vi "Axis Property to Cluster.vi"(11 "Axis Property Array In":T1[](array[typedef])) -> (3 "Axis Property Out":T2)   [LabVIEW 2020, in "3D Plot.lvclass"]
uses:
  <vilib>/Math Plots/3D Math Plots/3D Plot/3D Plot/3D Plot.lvclass
  <vilib>/Math Plots/3D Math Plots/3D Plot/3D Plot/Typedef/Axis Property.ctl
  <vilib>/Math Plots/3D Math Plots/3D Plot/3D Plot/Typedef/Caption Property.ctl
  <vilib>/Math Plots/3D Math Plots/3D Plot/3D Plot/Typedef/Label Property.ctl
  <vilib>/Math Plots/3D Math Plots/3D Plot/3D Plot/Typedef/Range Property.ctl
  <vilib>/Math Plots/3D Math Plots/3D Plot/3D Plot/Typedef/Range Clusters.ctl
  <vilib>/Math Plots/3D Math Plots/3D Plot/3D Plot/Typedef/Grid Property.ctl
  <vilib>/Math Plots/3D Math Plots/3D Plot/3D Plot/Typedef/Tick Property.ctl
  <vilib>/Math Plots/3D Math Plots/3D Plot/3D Plot/Typedef/Axis Property Array Element.ctl
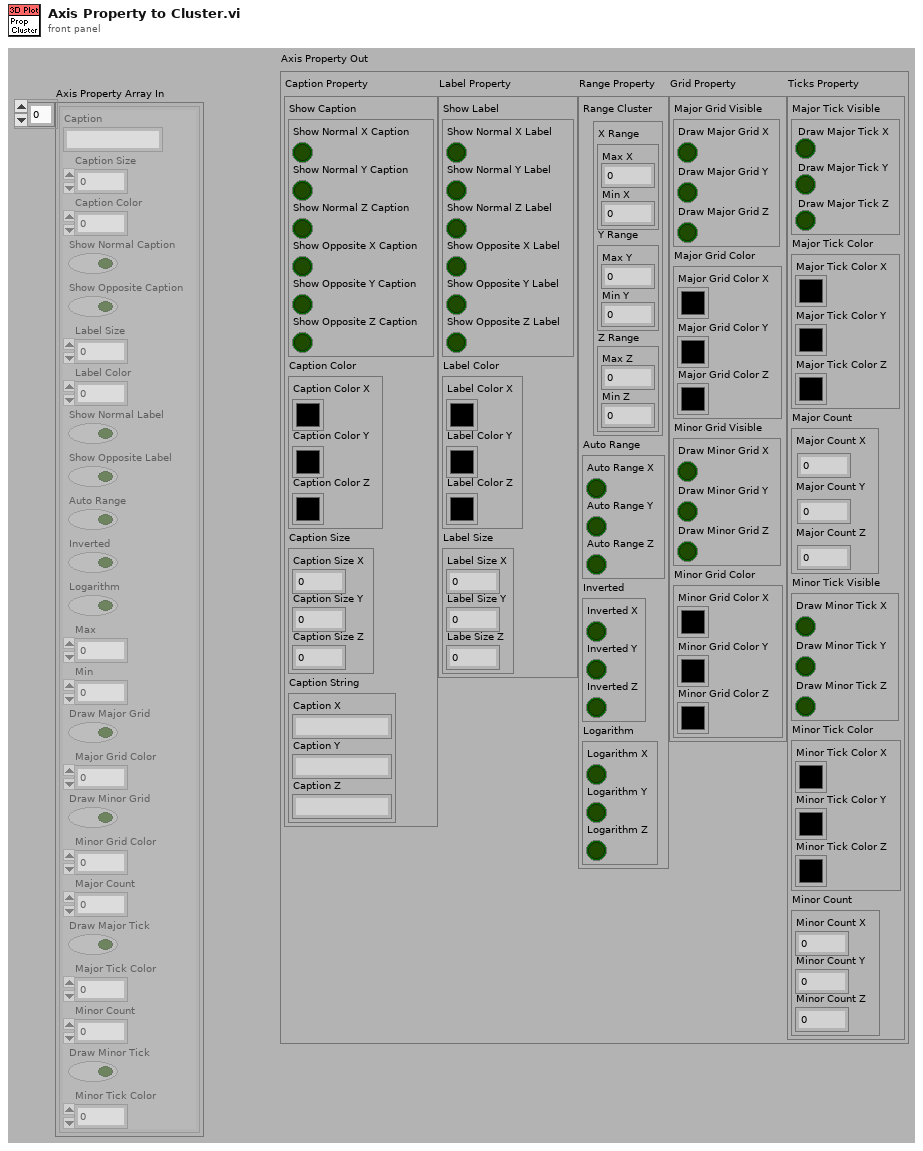
[diagram p1: front panel]
types:
  T1 = typedef "3D Plot.lvclass/Axis Property Array Element.ctl" = cluster{"Caption":string, "Caption Size":u16, "Caption Color":u32, "Show Normal Caption":bool, "Show Opposite Caption":bool, "Label Size":u16, "Label Color":u32, "Show Normal Label":bool, "Show Opposite Label":bool, "Auto Range":bool, "Inverted":bool, "Logarithm":bool, "Max":sgl, "Min":sgl, "Draw Major Grid":bool, "Major Grid Color":u32, "Draw Minor Grid":bool, "Minor Grid Color":u32, "Major Count":u16, "Draw Major Tick":bool, "Major Tick Color":u32, "Minor Count":u16, "Draw Minor Tick":bool, "Minor Tick Color":u32}
  T2 = typedef "3D Plot.lvclass/Axis Property.ctl" = cluster{"Caption Property":T3, "Label Property":T4, "Range Property":T5, "Grid Property":T7, "Ticks Property":T8}
  T3 = typedef "3D Plot.lvclass/Caption Property.ctl" = cluster{"Show Caption":cluster{"Show Normal X Caption":bool, "Show Normal Y Caption":bool, "Show Normal Z Caption":bool, "Show Opposite X Caption":bool, "Show Opposite Y Caption":bool, "Show Opposite Z Caption":bool}, "Caption Color":cluster{"Caption Color X":u32, "Caption Color Y":u32, "Caption Color Z":u32}, "Caption Size":cluster{"Caption Size X":u16, "Caption Size Y":u16, "Caption Size Z":u16}, "Caption String":cluster{"Caption X":string, "Caption Y":string, "Caption Z ":string}}
  T4 = typedef "3D Plot.lvclass/Label Property.ctl" = cluster{"Show Label":cluster{"Show Normal X Label":bool, "Show Normal Y Label":bool, "Show Normal Z Label":bool, "Show Opposite X Label":bool, "Show Opposite Y Label":bool, "Show Opposite Z Label":bool}, "Label Color":cluster{"Label Color X":u32, "Label Color Y":u32, "Label Color Z":u32}, "Label Size":cluster{"Label Size X":u16, "Label Size Y":u16, "Labe Size Z":u16}}
  T5 = typedef "3D Plot.lvclass/Range Property.ctl" = cluster{"Range Cluster":T6, "Auto Range":cluster{"Auto Range X":bool, "Auto Range Y":bool, "Auto Range Z":bool}, "Inverted":cluster{"Inverted X":bool, "Inverted Y":bool, "Inverted Z":bool}, "Logarithm":cluster{"Logarithm X":bool, "Logarithm Y":bool, "Logarithm Z":bool}}
  T6 = typedef "3D Plot.lvclass/Range Clusters.ctl" = cluster{"X Range":cluster{"Max X":sgl, "Min X":sgl}, "Y Range":cluster{"Max Y":sgl, "Min Y":sgl}, "Z Range":cluster{"Max Z":sgl, "Min Z":sgl}}
  T7 = typedef "3D Plot.lvclass/Grid Property.ctl" = cluster{"Major Grid Visible":cluster{"Draw Major Grid X":bool, "Draw Major Grid Y":bool, "Draw Major Grid Z":bool}, "Major Grid Color":cluster{"Major Grid Color X":u32, "Major Grid Color Y":u32, "Major Grid Color Z":u32}, "Minor Grid Visible":cluster{"Draw Minor Grid X":bool, "Draw Minor Grid Y":bool, "Draw Minor Grid Z":bool}, "Minor Grid Color":cluster{"Minor Grid Color X":u32, "Minor Grid Color Y":u32, "Minor Grid Color Z":u32}}
  T8 = typedef "3D Plot.lvclass/Tick Property.ctl" = cluster{"Major Tick Visible":cluster{"Draw Major Tick X":bool, "Draw Major Tick Y":bool, "Draw Major Tick Z":bool}, "Major Tick Color":cluster{"Major Tick Color X":u32, "Major Tick Color Y":u32, "Major Tick Color Z":u32}, "Major Count":cluster{"Major Count X":u16, "Major Count Y":u16, "Major Count Z":u16}, "Minor Tick Visible":cluster{"Draw Minor Tick X":bool, "Draw Minor Tick Y":bool, "Draw Minor Tick Z":bool}, "Minor Tick Color":cluster{"Minor Tick Color X":u32, "Minor Tick Color Y":u32, "Minor Tick Color Z":u32}, "Minor Count":cluster{"Minor Count X":u16, "Minor Count Y":u16, "Minor Count Z":u16}}
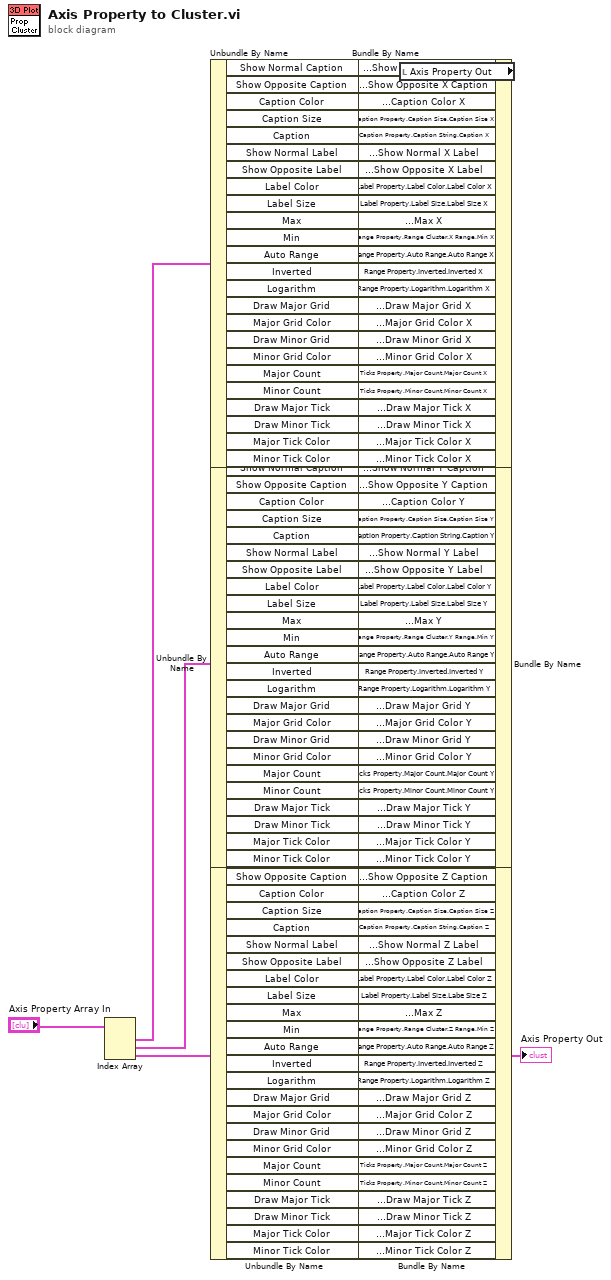
[diagram p0: block diagram]
diagram:
  n1 = Index Array(array="Axis Property Array In") -> (element #1=w79:T1, element #2=w54:T1, element #3=w53:T1)  [unwired: 3 in]
  n2 = Unbundle By Name(w79) -> ("Show Normal Caption"=w77:bool, "Show Opposite Caption"=w76:bool, "Caption Color"=w75:u32, "Caption Size"=w74:u16, "Caption"=w73:string, "Show Normal Label"=w72:bool, "Show Opposite Label"=w71:bool, "Label Color"=w70:u32, "Label Size"=w69:u16, "Max"=w68:sgl, "Min"=w67:sgl, "Auto Range"=w66:bool, "Inverted"=w65:bool, "Logarithm"=w3:bool, "Draw Major Grid"=w64:bool, "Major Grid Color"=w63:u32, "Draw Minor Grid"=w62:bool, "Minor Grid Color"=w61:u32, "Major Count"=w60:u16, "Minor Count"=w59:u16, "Draw Major Tick"=w58:bool, "Draw Minor Tick"=w57:bool, "Major Tick Color"=w56:u32, "Minor Tick Color"=w55:u32)
  n3 = Unbundle By Name(w54) -> ("Show Normal Caption"=w49:bool, "Show Opposite Caption"=w48:bool, "Caption Color"=w47:u32, "Caption Size"=w46:u16, "Caption"=w45:string, "Show Normal Label"=w44:bool, "Show Opposite Label"=w43:bool, "Label Color"=w42:u32, "Label Size"=w41:u16, "Max"=w40:sgl, "Min"=w39:sgl, "Auto Range"=w38:bool, "Inverted"=w37:bool, "Logarithm"=w2:bool, "Draw Major Grid"=w36:bool, "Major Grid Color"=w35:u32, "Draw Minor Grid"=w34:bool, "Minor Grid Color"=w33:u32, "Major Count"=w32:u16, "Minor Count"=w31:u16, "Draw Major Tick"=w30:bool, "Draw Minor Tick"=w29:bool, "Major Tick Color"=w28:u32, "Minor Tick Color"=w27:u32)
  n4 = Unbundle By Name(w53) -> ("Show Normal Caption"=w26:bool, "Show Opposite Caption"=w25:bool, "Caption Color"=w24:u32, "Caption Size"=w23:u16, "Caption"=w21:string, "Show Normal Label"=w22:bool, "Show Opposite Label"=w20:bool, "Label Color"=w19:u32, "Label Size"=w18:u16, "Max"=w17:sgl, "Min"=w15:sgl, "Auto Range"=w16:bool, "Inverted"=w14:bool, "Logarithm"=w1:bool, "Draw Major Grid"=w13:bool, "Major Grid Color"=w12:u32, "Draw Minor Grid"=w11:bool, "Minor Grid Color"=w10:u32, "Major Count"=w9:u16, "Minor Count"=w8:u16, "Draw Major Tick"=w7:bool, "Draw Minor Tick"=w6:bool, "Major Tick Color"=w5:u32, "Minor Tick Color"=w4:u32)
  n5 = local read "Axis Property Out"() -> (w78:T2)
  n6 = Bundle By Name(cluster=w78, "Caption Property.Show Caption.Show Normal X Caption"=w77, "Caption Property.Show Caption.Show Opposite X Caption"=w76, "Caption Property.Caption Color.Caption Color X"=w75, "Caption Property.Caption Size.Caption Size X"=w74, "Caption Property.Caption String.Caption X"=w73, "Label Property.Show Label.Show Normal X Label"=w72, "Label Property.Show Label.Show Opposite X Label"=w71, "Label Property.Label Color.Label Color X"=w70, "Label Property.Label Size.Label Size X"=w69, "Range Property.Range Cluster.X Range.Max X"=w68, "Range Property.Range Cluster.X Range.Min X"=w67, "Range Property.Auto Range.Auto Range X"=w66, "Range Property.Inverted.Inverted X"=w65, "Range Property.Logarithm.Logarithm X"=w3, "Grid Property.Major Grid Visible.Draw Major Grid X"=w64, "Grid Property.Major Grid Color.Major Grid Color X"=w63, "Grid Property.Minor Grid Visible.Draw Minor Grid X"=w62, "Grid Property.Minor Grid Color.Minor Grid Color X"=w61, "Ticks Property.Major Count.Major Count X"=w60, "Ticks Property.Minor Count.Minor Count X"=w59, "Ticks Property.Major Tick Visible.Draw Major Tick X"=w58, "Ticks Property.Minor Tick Visible.Draw Minor Tick X"=w57, "Ticks Property.Major Tick Color.Major Tick Color X"=w56, "Ticks Property.Minor Tick Color.Minor Tick Color X"=w55) -> (w52:T2)
  n7 = Bundle By Name(cluster=w52, "Caption Property.Show Caption.Show Normal Y Caption"=w49, "Caption Property.Show Caption.Show Opposite Y Caption"=w48, "Caption Property.Caption Color.Caption Color Y"=w47, "Caption Property.Caption Size.Caption Size Y"=w46, "Caption Property.Caption String.Caption Y"=w45, "Label Property.Show Label.Show Normal Y Label"=w44, "Label Property.Show Label.Show Opposite Y Label"=w43, "Label Property.Label Color.Label Color Y"=w42, "Label Property.Label Size.Label Size Y"=w41, "Range Property.Range Cluster.Y Range.Max Y"=w40, "Range Property.Range Cluster.Y Range.Min Y"=w39, "Range Property.Auto Range.Auto Range Y"=w38, "Range Property.Inverted.Inverted Y"=w37, "Range Property.Logarithm.Logarithm Y"=w2, "Grid Property.Major Grid Visible.Draw Major Grid Y"=w36, "Grid Property.Major Grid Color.Major Grid Color Y"=w35, "Grid Property.Minor Grid Visible.Draw Minor Grid Y"=w34, "Grid Property.Minor Grid Color.Minor Grid Color Y"=w33, "Ticks Property.Major Count.Major Count Y"=w32, "Ticks Property.Minor Count.Minor Count Y"=w31, "Ticks Property.Major Tick Visible.Draw Major Tick Y"=w30, "Ticks Property.Minor Tick Visible.Draw Minor Tick Y"=w29, "Ticks Property.Major Tick Color.Major Tick Color Y"=w28, "Ticks Property.Minor Tick Color.Minor Tick Color Y"=w27) -> (w51:T2)
  n8 = Bundle By Name(cluster=w51, "Caption Property.Show Caption.Show Normal Z Caption"=w26, "Caption Property.Show Caption.Show Opposite Z Caption"=w25, "Caption Property.Caption Color.Caption Color Z"=w24, "Caption Property.Caption Size.Caption Size Z"=w23, "Caption Property.Caption String.Caption Z"=w21, "Label Property.Show Label.Show Normal Z Label"=w22, "Label Property.Show Label.Show Opposite Z Label"=w20, "Label Property.Label Color.Label Color Z"=w19, "Label Property.Label Size.Labe Size Z"=w18, "Range Property.Range Cluster.Z Range.Max Z"=w17, "Range Property.Range Cluster.Z Range.Min Z"=w15, "Range Property.Auto Range.Auto Range Z"=w16, "Range Property.Inverted.Inverted Z"=w14, "Range Property.Logarithm.Logarithm Z"=w1, "Grid Property.Major Grid Visible.Draw Major Grid Z"=w13, "Grid Property.Major Grid Color.Major Grid Color Z"=w12, "Grid Property.Minor Grid Visible.Draw Minor Grid Z"=w11, "Grid Property.Minor Grid Color.Minor Grid Color Z"=w10, "Ticks Property.Major Count.Major Count Z"=w9, "Ticks Property.Minor Count.Minor Count Z"=w8, "Ticks Property.Major Tick Visible.Draw Major Tick Z"=w7, "Ticks Property.Minor Tick Visible.Draw Minor Tick Z"=w6, "Ticks Property.Major Tick Color.Major Tick Color Z"=w5, "Ticks Property.Minor Tick Color.Minor Tick Color Z"=w4) -> (→"Axis Property Out":T2)
